vi "Set Log File Archive Location.vi"(8 "error in (no error)":errorcluster, 9 "archive directory parts":string[](array[string]), 10 "archive closed log files":bool, 11 "log file in":T1 format="%.0x") -> (0 "error out":errorcluster, 3 "log file out":T1 format="%.0x")   [LabVIEW 2027, in "Embedded Data Logger Scripting.lvlib"]
uses:
  Embedded Data Logger Scripting.lvlib
  <vilib>/NI VeriStand/Custom Device API/Custom Device Item Ref.ctl
  Shared/Constants.vi
  <vilib>/NI VeriStand/Custom Device API/Set Item Property (Boolean).vi
  <vilib>/NI VeriStand/Custom Device API/Set Item Property (String Array).vi
  Shared/Embedded Data Logger Shared.lvlib
  <vilib>/NI VeriStand/Custom Device API/Custom Device API.lvlib
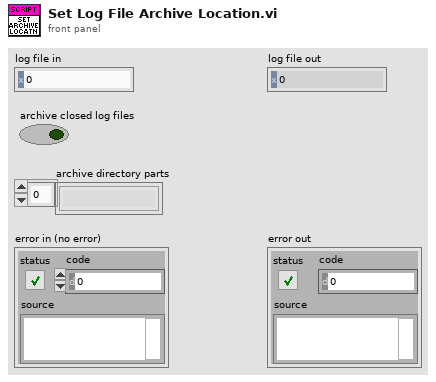
[diagram p1: front panel]
types:
  T1 = typedef "Custom Device API.lvlib/Custom Device Item Ref.ctl" = u64
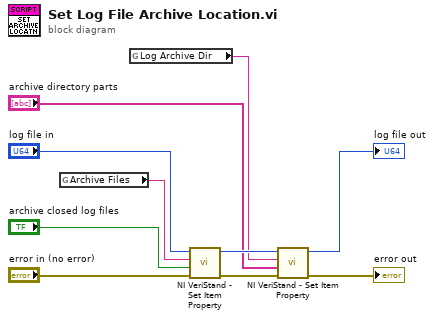
[diagram p0: block diagram]
diagram:
  n1 = global read "Constants.vi" "Archive Files"() -> (w5:string)
  n2 = global read "Constants.vi" "Log Archive Dir"() -> (w1:string)
  n3 = call-poly <vilib>:"NI VeriStand - Set Item Property.vi"("error in (no error)"="error in (no error)", "Value"="archive closed log files", "Property Name"=w5, "Item Ref in"="log file in") -> ("error out"=w7:errorcluster, "Item Ref out"=w8:T1)  [unwired: 5 in, 1 out]
  n4 = call-poly <vilib>:"NI VeriStand - Set Item Property.vi"("error in (no error)"=w7, "Value"="archive directory parts", "Property Name"=w1, "Item Ref in"=w8) -> ("error out"=→"error out":errorcluster, "Item Ref out"=→"log file out":T1)  [unwired: 5 in, 1 out]
